vi "LV Demo Main.vi"() -> ()   [LabVIEW 2017, in "Powermeter_library.lvlib"]
uses:
  Powermeter_library.lvlib
  Channel States.ctl
  <vilib>/regexp/Match Regular Expression.xnode
panel:
  out "File Size":i64=76
  in  "Tab Control":enum32{"File", "Page 2"}(tab)
  in  "Filename":string="Run1_Powermeter"
  out "file path":path=path "E:/HVOF - Tests/2017/Recombination/2017-10-04/Run1_Powermeter.tdms"
  in  "base path":path=path "E:/HVOF - Tests/2017/Recombination"
  in  "Group name append":string
  in  "Meas On":bool[](array[boolean])=[TRUE]
  in  "scan again":bool=TRUE
  in  "All Handles":i32[](array[numeric])=[1000]
  in  "Get Lib Ver":bool
  in  "Get Driver Ver":bool
  out "LibVer":i32
  out "DriverVer":string
  out "output cluster":T1
  in  "Reset graph 2":bool
  out "Timestamp offset":dbl
  out "First Data point":bool=TRUE
  out "Power meter 2":cluster{timestamp[], dbl[]}(graph)={[timestamp(3586444920.089349 s since 1904-01-01), timestamp(3586444920.2053604 s since 1904-01-01), timestamp(3586444920.2613664 s since 1904-01-01), timestamp(3586444920.370377 s since 1904-01-01), timestamp(3586444920.479388 s since 1904-01-01), timestamp(3586444920.588399 s since 1904-01-01), timestamp(3586444920.70241 s since 1904-01-01), timestamp(3586444920.7584157 s since 1904-01-01), timestamp(3586444920.868427 s since 1904-01-01), timestamp(3586444920.978438 s since 1904-01-01), timestamp(3586444921.0864487 s since 1904-01-01), timestamp(3586444921.19646 s since 1904-01-01), timestamp(3586444921.253465 s since 1904-01-01), timestamp(3586444921.3664765 s since 1904-01-01), timestamp(3586444921.6875086 s since 1904-01-01), timestamp(3586444921.7935195 s since 1904-01-01), timestamp(3586444922.0625463 s since 1904-01-01), timestamp(3586444922.170557 s since 1904-01-01), timestamp(3586444922.491589 s since 1904-01-01), timestamp(3586444922.6016 s since 1904-01-01), timestamp(3586444922.868627 s since 1904-01-01), timestamp(3586444922.977638 s since 1904-01-01), timestamp(3586444923.29867 s since 1904-01-01), timestamp(3586444923.3546753 s since 1904-01-01), timestamp(3586444923.6767077 s since 1904-01-01), timestamp(3586444923.7857184 s since 1904-01-01), timestamp(3586444924.0537453 s since 1904-01-01), timestamp(3586444924.161756 s since 1904-01-01), timestamp(3586444924.270767 s since 1904-01-01), timestamp(3586444924.379778 s since 1904-01-01), timestamp(3586444924.489789 s since 1904-01-01), timestamp(3586444924.6028004 s since 1904-01-01), timestamp(3586444924.6558056 s since 1904-01-01), timestamp(3586444924.772817 s since 1904-01-01), timestamp(3586444924.880828 s since 1904-01-01), timestamp(3586444924.952835 s since 1904-01-01), timestamp(3586444925.062846 s since 1904-01-01), timestamp(3586444925.168857 s since 1904-01-01), timestamp(3586444925.2788677 s since 1904-01-01), timestamp(3586444925.3868785 s since 1904-01-01), timestamp(3586444925.4968896 s since 1904-01-01), timestamp(3586444925.552895 s since 1904-01-01), timestamp(3586444925.6619062 s since 1904-01-01), timestamp(3586444925.770917 s since 1904-01-01), timestamp(3586444925.879928 s since 1904-01-01), timestamp(3586444925.987939 s since 1904-01-01), timestamp(3586444926.0939493 s since 1904-01-01), timestamp(3586444926.149955 s since 1904-01-01), timestamp(3586444926.2609663 s since 1904-01-01), timestamp(3586444926.370977 s since 1904-01-01), timestamp(3586444926.479988 s since 1904-01-01), timestamp(3586444926.588999 s since 1904-01-01), timestamp(3586444926.69801 s since 1904-01-01), timestamp(3586444926.7540154 s since 1904-01-01), timestamp(3586444926.863026 s since 1904-01-01), timestamp(3586444926.9760375 s since 1904-01-01), timestamp(3586444927.0850487 s since 1904-01-01), timestamp(3586444927.191059 s since 1904-01-01), timestamp(3586444927.30207 s since 1904-01-01), timestamp(3586444927.356076 s since 1904-01-01), timestamp(3586444927.4650865 s since 1904-01-01), timestamp(3586444927.5790977 s since 1904-01-01), timestamp(3586444927.688109 s since 1904-01-01), timestamp(3586444927.849125 s since 1904-01-01), timestamp(3586444927.9581356 s since 1904-01-01), timestamp(3586444928.0681467 s since 1904-01-01), timestamp(3586444928.180158 s since 1904-01-01), timestamp(3586444928.289169 s since 1904-01-01), timestamp(3586444928.39818 s since 1904-01-01), timestamp(3586444928.4661865 s since 1904-01-01), timestamp(3586444928.581198 s since 1904-01-01), timestamp(3586444928.6942096 s since 1904-01-01), timestamp(3586444928.750215 s since 1904-01-01), timestamp(3586444928.870227 s since 1904-01-01), timestamp(3586444928.9772377 s since 1904-01-01), timestamp(3586444929.0932493 s since 1904-01-01), timestamp(3586444929.149255 s since 1904-01-01), timestamp(3586444929.259266 s since 1904-01-01), timestamp(3586444929.3672767 s since 1904-01-01), timestamp(3586444929.4762874 s since 1904-01-01), timestamp(3586444929.5852985 s since 1904-01-01), timestamp(3586444929.694309 s since 1904-01-01), timestamp(3586444929.750315 s since 1904-01-01), timestamp(3586444929.862326 s since 1904-01-01), timestamp(3586444929.9763374 s since 1904-01-01), timestamp(3586444930.0863485 s since 1904-01-01), timestamp(3586444930.1943593 s since 1904-01-01), timestamp(3586444930.249365 s since 1904-01-01), timestamp(3586444930.358376 s since 1904-01-01), timestamp(3586444930.4763875 s since 1904-01-01), timestamp(3586444930.5853987 s since 1904-01-01), timestamp(3586444930.6944094 s since 1904-01-01), timestamp(3586444930.7514153 s since 1904-01-01), timestamp(3586444930.859426 s since 1904-01-01), timestamp(3586444930.9654365 s since 1904-01-01), timestamp(3586444931.0754476 s since 1904-01-01), timestamp(3586444931.190459 s since 1904-01-01), timestamp(3586444931.29947 s since 1904-01-01), timestamp(3586444931.3554754 s since 1904-01-01), timestamp(3586444931.4644866 s since 1904-01-01), timestamp(3586444931.7845182 s since 1904-01-01), timestamp(3586444931.8935294 s since 1904-01-01), timestamp(3586444931.949535 s since 1904-01-01), timestamp(3586444932.059546 s since 1904-01-01), timestamp(3586444932.1685567 s since 1904-01-01), timestamp(3586444932.277568 s since 1904-01-01), timestamp(3586444932.3875785 s since 1904-01-01), timestamp(3586444932.4965897 s since 1904-01-01), timestamp(3586444932.552595 s since 1904-01-01), timestamp(3586444932.6616063 s since 1904-01-01), timestamp(3586444932.770617 s since 1904-01-01), timestamp(3586444932.8796277 s since 1904-01-01), timestamp(3586444932.9866385 s since 1904-01-01), timestamp(3586444933.0956497 s since 1904-01-01), timestamp(3586444933.151655 s since 1904-01-01), timestamp(3586444933.2616663 s since 1904-01-01), timestamp(3586444933.374677 s since 1904-01-01), timestamp(3586444933.4836884 s since 1904-01-01), timestamp(3586444933.592699 s since 1904-01-01), timestamp(3586444933.649705 s since 1904-01-01), timestamp(3586444933.7587156 s since 1904-01-01), timestamp(3586444933.8667264 s since 1904-01-01), timestamp(3586444933.9757376 s since 1904-01-01), timestamp(3586444934.0837483 s since 1904-01-01), timestamp(3586444934.191759 s since 1904-01-01), timestamp(3586444934.29977 s since 1904-01-01), timestamp(3586444934.3557754 s since 1904-01-01), timestamp(3586444934.4647865 s since 1904-01-01), timestamp(3586444934.573797 s since 1904-01-01), timestamp(3586444934.6828084 s since 1904-01-01), timestamp(3586444934.791819 s since 1904-01-01), timestamp(3586444934.89883 s since 1904-01-01), timestamp(3586444934.9548354 s since 1904-01-01), timestamp(3586444935.063846 s since 1904-01-01), timestamp(3586444935.171857 s since 1904-01-01), timestamp(3586444935.280868 s since 1904-01-01), timestamp(3586444935.3898787 s since 1904-01-01), timestamp(3586444935.49989 s since 1904-01-01), timestamp(3586444935.5568957 s since 1904-01-01), timestamp(3586444935.6659064 s since 1904-01-01), timestamp(3586444935.770917 s since 1904-01-01), timestamp(3586444935.879928 s since 1904-01-01), timestamp(3586444935.988939 s since 1904-01-01), timestamp(3586444936.0979495 s since 1904-01-01), timestamp(3586444936.1539555 s since 1904-01-01), timestamp(3586444936.261966 s since 1904-01-01), timestamp(3586444936.370977 s since 1904-01-01), timestamp(3586444936.479988 s since 1904-01-01), timestamp(3586444936.588999 s since 1904-01-01), timestamp(3586444936.69901 s since 1904-01-01), timestamp(3586444936.7550154 s since 1904-01-01), timestamp(3586444936.864026 s since 1904-01-01), timestamp(3586444936.9720373 s since 1904-01-01), timestamp(3586444937.081048 s since 1904-01-01), timestamp(3586444937.189059 s since 1904-01-01), timestamp(3586444937.29907 s since 1904-01-01), timestamp(3586444937.3550754 s since 1904-01-01), timestamp(3586444937.4640865 s since 1904-01-01), timestamp(3586444937.573097 s since 1904-01-01), timestamp(3586444937.6831083 s since 1904-01-01)], [0.0, 0.0, 0.0, 0.0, 0.0, 0.0, 0.0, 0.0, 0.0, 0.0, 0.0, 0.0, 0.0, 0.0, 0.0, 0.0, 0.0, 0.0, 0.0, 0.0, 0.0, 0.0, 0.0, 0.0, 0.0, 0.0, 0.0, 0.0, 0.0, 0.0, 0.0, 0.0, 0.0, 0.0, 0.0, 0.0, 0.0, 0.0, 0.0, 0.0, 0.0, 0.0, 0.0, 0.0, 0.0, 0.0, 0.0, 0.0, 0.0, 0.0, 0.0, 0.0, 0.0, 0.0, 0.0, 0.0, 0.0, 0.0, 0.0, 0.0, 0.0, 0.0, 0.0, 0.0, 0.0, 0.0, 0.0, 0.0, 0.0, 0.0, 0.0, 0.0, 0.0, 0.0, 0.0, 0.0, 0.0, 0.0, 0.0, 0.0, 0.0, 0.0, 0.0, 0.0, 0.0, 0.0, 0.0, 0.0, 0.0, 0.0, 0.0, 0.0, 0.0, 0.0, 0.0, 0.0, 0.0, 0.0, 0.0, 0.0, 0.0, 0.0, 0.0, 0.0, 0.0, 0.0, 0.0, 0.0, 0.0, 0.0, 0.0, 0.0, 0.0, 0.0, 0.0, 0.0, 0.0, 0.0, 0.0, 0.0, 0.0, 0.0, 0.0, 0.0, 0.0, 0.0, 0.0, 0.0, 0.0, 0.0, 0.0, 0.0, 0.0, 0.0, 0.0, 0.0, 0.0, 0.0, 0.0, 0.0, 0.0, 0.0, 0.0, 0.0, 0.0, 0.0, 0.0, 0.0, 0.0, 0.0, 0.0, 0.0, 0.0, 0.0, 0.0, 0.0, 0.0, 0.0, 0.0, 0.0]}
  in  "Reset graph 1":bool
  out "TDMS error":errorcluster
  out "TDMS file":refnum<k34>
  out "Power meter 1":cluster{timestamp[], dbl[]}(graph)={[timestamp(3586444920.089349 s since 1904-01-01), timestamp(3586444920.2053604 s since 1904-01-01), timestamp(3586444920.2613664 s since 1904-01-01), timestamp(3586444920.370377 s since 1904-01-01), timestamp(3586444920.479388 s since 1904-01-01), timestamp(3586444920.588399 s since 1904-01-01), timestamp(3586444920.70241 s since 1904-01-01), timestamp(3586444920.7584157 s since 1904-01-01), timestamp(3586444920.868427 s since 1904-01-01), timestamp(3586444920.978438 s since 1904-01-01), timestamp(3586444921.0864487 s since 1904-01-01), timestamp(3586444921.19646 s since 1904-01-01), timestamp(3586444921.253465 s since 1904-01-01), timestamp(3586444921.3664765 s since 1904-01-01), timestamp(3586444921.6875086 s since 1904-01-01), timestamp(3586444921.7935195 s since 1904-01-01), timestamp(3586444922.0625463 s since 1904-01-01), timestamp(3586444922.170557 s since 1904-01-01), timestamp(3586444922.491589 s since 1904-01-01), timestamp(3586444922.6016 s since 1904-01-01), timestamp(3586444922.868627 s since 1904-01-01), timestamp(3586444922.977638 s since 1904-01-01), timestamp(3586444923.29867 s since 1904-01-01), timestamp(3586444923.3546753 s since 1904-01-01), timestamp(3586444923.6767077 s since 1904-01-01), timestamp(3586444923.7857184 s since 1904-01-01), timestamp(3586444924.0537453 s since 1904-01-01), timestamp(3586444924.161756 s since 1904-01-01), timestamp(3586444924.270767 s since 1904-01-01), timestamp(3586444924.379778 s since 1904-01-01), timestamp(3586444924.489789 s since 1904-01-01), timestamp(3586444924.6028004 s since 1904-01-01), timestamp(3586444924.6558056 s since 1904-01-01), timestamp(3586444924.772817 s since 1904-01-01), timestamp(3586444924.880828 s since 1904-01-01), timestamp(3586444924.952835 s since 1904-01-01), timestamp(3586444925.062846 s since 1904-01-01), timestamp(3586444925.168857 s since 1904-01-01), timestamp(3586444925.2788677 s since 1904-01-01), timestamp(3586444925.3868785 s since 1904-01-01), timestamp(3586444925.4968896 s since 1904-01-01), timestamp(3586444925.552895 s since 1904-01-01), timestamp(3586444925.6619062 s since 1904-01-01), timestamp(3586444925.770917 s since 1904-01-01), timestamp(3586444925.879928 s since 1904-01-01), timestamp(3586444925.987939 s since 1904-01-01), timestamp(3586444926.0939493 s since 1904-01-01), timestamp(3586444926.149955 s since 1904-01-01), timestamp(3586444926.2609663 s since 1904-01-01), timestamp(3586444926.370977 s since 1904-01-01), timestamp(3586444926.479988 s since 1904-01-01), timestamp(3586444926.588999 s since 1904-01-01), timestamp(3586444926.69801 s since 1904-01-01), timestamp(3586444926.7540154 s since 1904-01-01), timestamp(3586444926.863026 s since 1904-01-01), timestamp(3586444926.9760375 s since 1904-01-01), timestamp(3586444927.0850487 s since 1904-01-01), timestamp(3586444927.191059 s since 1904-01-01), timestamp(3586444927.30207 s since 1904-01-01), timestamp(3586444927.356076 s since 1904-01-01), timestamp(3586444927.4650865 s since 1904-01-01), timestamp(3586444927.5790977 s since 1904-01-01), timestamp(3586444927.688109 s since 1904-01-01), timestamp(3586444927.849125 s since 1904-01-01), timestamp(3586444927.9581356 s since 1904-01-01), timestamp(3586444928.0681467 s since 1904-01-01), timestamp(3586444928.180158 s since 1904-01-01), timestamp(3586444928.289169 s since 1904-01-01), timestamp(3586444928.39818 s since 1904-01-01), timestamp(3586444928.4661865 s since 1904-01-01), timestamp(3586444928.581198 s since 1904-01-01), timestamp(3586444928.6942096 s since 1904-01-01), timestamp(3586444928.750215 s since 1904-01-01), timestamp(3586444928.870227 s since 1904-01-01), timestamp(3586444928.9772377 s since 1904-01-01), timestamp(3586444929.0932493 s since 1904-01-01), timestamp(3586444929.149255 s since 1904-01-01), timestamp(3586444929.259266 s since 1904-01-01), timestamp(3586444929.3672767 s since 1904-01-01), timestamp(3586444929.4762874 s since 1904-01-01), timestamp(3586444929.5852985 s since 1904-01-01), timestamp(3586444929.694309 s since 1904-01-01), timestamp(3586444929.750315 s since 1904-01-01), timestamp(3586444929.862326 s since 1904-01-01), timestamp(3586444929.9763374 s since 1904-01-01), timestamp(3586444930.0863485 s since 1904-01-01), timestamp(3586444930.1943593 s since 1904-01-01), timestamp(3586444930.249365 s since 1904-01-01), timestamp(3586444930.358376 s since 1904-01-01), timestamp(3586444930.4763875 s since 1904-01-01), timestamp(3586444930.5853987 s since 1904-01-01), timestamp(3586444930.6944094 s since 1904-01-01), timestamp(3586444930.7514153 s since 1904-01-01), timestamp(3586444930.859426 s since 1904-01-01), timestamp(3586444930.9654365 s since 1904-01-01), timestamp(3586444931.0754476 s since 1904-01-01), timestamp(3586444931.190459 s since 1904-01-01), timestamp(3586444931.29947 s since 1904-01-01), timestamp(3586444931.3554754 s since 1904-01-01), timestamp(3586444931.4644866 s since 1904-01-01), timestamp(3586444931.7845182 s since 1904-01-01), timestamp(3586444931.8935294 s since 1904-01-01), timestamp(3586444931.949535 s since 1904-01-01), timestamp(3586444932.059546 s since 1904-01-01), timestamp(3586444932.1685567 s since 1904-01-01), timestamp(3586444932.277568 s since 1904-01-01), timestamp(3586444932.3875785 s since 1904-01-01), timestamp(3586444932.4965897 s since 1904-01-01), timestamp(3586444932.552595 s since 1904-01-01), timestamp(3586444932.6616063 s since 1904-01-01), timestamp(3586444932.770617 s since 1904-01-01), timestamp(3586444932.8796277 s since 1904-01-01), timestamp(3586444932.9866385 s since 1904-01-01), timestamp(3586444933.0956497 s since 1904-01-01), timestamp(3586444933.151655 s since 1904-01-01), timestamp(3586444933.2616663 s since 1904-01-01), timestamp(3586444933.374677 s since 1904-01-01), timestamp(3586444933.4836884 s since 1904-01-01), timestamp(3586444933.592699 s since 1904-01-01), timestamp(3586444933.649705 s since 1904-01-01), timestamp(3586444933.7587156 s since 1904-01-01), timestamp(3586444933.8667264 s since 1904-01-01), timestamp(3586444933.9757376 s since 1904-01-01), timestamp(3586444934.0837483 s since 1904-01-01), timestamp(3586444934.191759 s since 1904-01-01), timestamp(3586444934.29977 s since 1904-01-01), timestamp(3586444934.3557754 s since 1904-01-01), timestamp(3586444934.4647865 s since 1904-01-01), timestamp(3586444934.573797 s since 1904-01-01), timestamp(3586444934.6828084 s since 1904-01-01), timestamp(3586444934.791819 s since 1904-01-01), timestamp(3586444934.89883 s since 1904-01-01), timestamp(3586444934.9548354 s since 1904-01-01), timestamp(3586444935.063846 s since 1904-01-01), timestamp(3586444935.171857 s since 1904-01-01), timestamp(3586444935.280868 s since 1904-01-01), timestamp(3586444935.3898787 s since 1904-01-01), timestamp(3586444935.49989 s since 1904-01-01), timestamp(3586444935.5568957 s since 1904-01-01), timestamp(3586444935.6659064 s since 1904-01-01), timestamp(3586444935.770917 s since 1904-01-01), timestamp(3586444935.879928 s since 1904-01-01), timestamp(3586444935.988939 s since 1904-01-01), timestamp(3586444936.0979495 s since 1904-01-01), timestamp(3586444936.1539555 s since 1904-01-01), timestamp(3586444936.261966 s since 1904-01-01), timestamp(3586444936.370977 s since 1904-01-01), timestamp(3586444936.479988 s since 1904-01-01), timestamp(3586444936.588999 s since 1904-01-01), timestamp(3586444936.69901 s since 1904-01-01), timestamp(3586444936.7550154 s since 1904-01-01), timestamp(3586444936.864026 s since 1904-01-01), timestamp(3586444936.9720373 s since 1904-01-01), timestamp(3586444937.081048 s since 1904-01-01), timestamp(3586444937.189059 s since 1904-01-01), timestamp(3586444937.29907 s since 1904-01-01), timestamp(3586444937.3550754 s since 1904-01-01), timestamp(3586444937.4640865 s since 1904-01-01), timestamp(3586444937.573097 s since 1904-01-01), timestamp(3586444937.6831083 s since 1904-01-01)], [0.0, 0.0, 0.0, 0.0, 0.0, 0.0, 0.0, 0.0, 0.0, 0.0, 0.0, 0.0, 0.0, 0.0, 0.0, 0.0, 0.0, 0.0, 0.0, 0.0, 0.0, 0.0, 0.0, 0.0, 0.0, 0.0, 0.0, 0.0, 0.0, 0.0, 0.0, 0.0, 0.0, 0.0, 0.0, 0.0, 0.0, 0.0, 0.0, 0.0, 0.0, 0.0, 0.0, 0.0, 0.0, 0.0, 0.0, 0.0, 0.0, 0.0, 0.0, 0.0, 0.0, 0.0, 0.0, 0.0, 0.0, 0.0, 0.0, 0.0, 0.0, 0.0, 0.0, 0.0, 0.0, 0.0, 0.0, 0.0, 0.0, 0.0, 0.0, 0.0, 0.0, 0.0, 0.0, 0.0, 0.0, 0.0, 0.0, 0.0, 0.0, 0.0, 0.0, 0.0, 0.0, 0.0, 0.0, 0.0, 0.0, 0.0, 0.0, 0.0, 0.0, 0.0, 0.0, 0.0, 0.0, 0.0, 0.0, 0.0, 0.0, 0.0, 0.0, 0.0, 0.0, 0.0, 0.0, 0.0, 0.0, 0.0, 0.0, 0.0, 0.0, 0.0, 0.0, 0.0, 0.0, 0.0, 0.0, 0.0, 0.0, 0.0, 0.0, 0.0, 0.0, 0.0, 0.0, 0.0, 0.0, 0.0, 0.0, 0.0, 0.0, 0.0, 0.0, 0.0, 0.0, 0.0, 0.0, 0.0, 0.0, 0.0, 0.0, 0.0, 0.0, 0.0, 0.0, 0.0, 0.0, 0.0, 0.0, 0.0, 0.0, 0.0, 0.0, 0.0, 0.0, 0.0, 0.0, 0.0]}
  in  "Save data":bool=TRUE
  in  "Stop":bool
  out "ReadStr":string
  in  "Read/Write":T2
  out "Device Name":string="(0)"
  in  "Dev Control":T3 {"externTrigModes" items=["Rising Edge", "Falling Edge", "High Level", "Low Level", "Output High", "Output Low"]; "Stream Modes:" items=["Turbo", "Turbo Freq", "Immediate"]}
  out "Last Error Code:":string="No Error"
  in  "Gen'l Ops":T4
  # "Local variables"
  # "v1.14"
  # "Write / Read"
  # "Device Control"
  # "Streams:"
  # "Ext Trig::"
  # "Device Management"
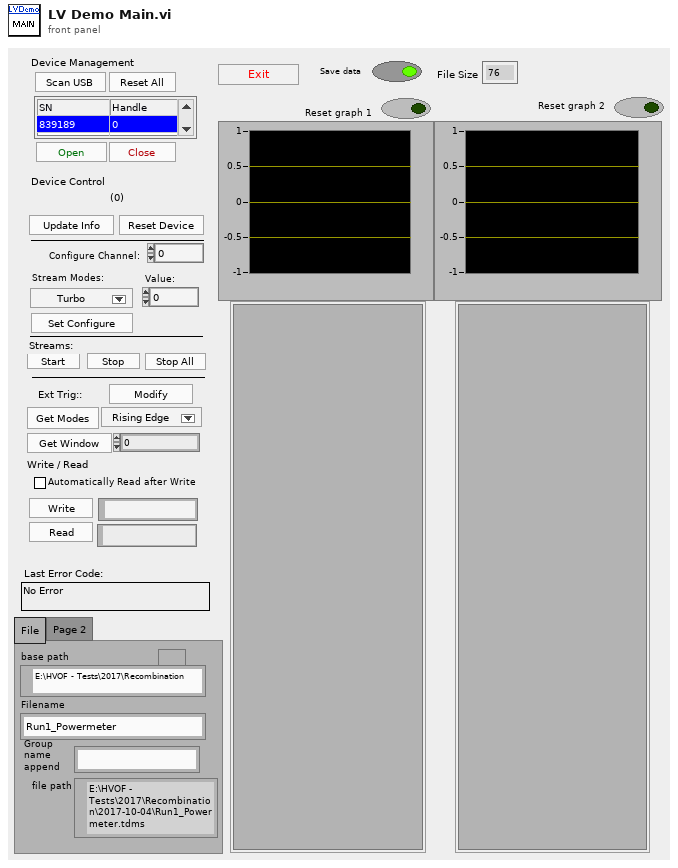
[diagram p1: front panel]
types:
  T1 = cluster{"output cluster 2":cluster{"Value:":dbl[], timestamp[], string[][]}, "output cluster 3":cluster{"Value:":dbl[], timestamp[], string[][]}}
  T2 = cluster{"AutoRead":bool, "Write":bool, "Read":bool, "WriteStr":string}
  T3 = cluster{"UpdateInfo":bool, "ResetDev":bool, "ConfigCh":i32, "Stream Modes:":i32, "Value":i32, "SetConfig":bool, "StartStream":bool, "StopStream":bool, "StopAll":bool, "externTrigModes":i32, "GetModes":bool, "GetWindow":bool, "ExtTrig Window":i32, "Modify":bool}
  T4 = cluster{"scanUSB":bool, "Devices":i32, "Open":bool, "Close":bool, "ResetAll":bool}
  T5 = cluster{"Value:":dbl[], " Time:":string[], " Status:":string[]}
  T6 = enum32{"invalid app kind", "Development System", "Run Time System", "Student Edition", "Embedded LabVIEW", "Evaluation", "Custom"}
  T7 = cluster{"Value:":dbl[], " Time:":string[], " Status:":string[]}[]
  T8 = typedef "Powermeter_library.lvlib/Channel States.ctl" = enum16{"Init", "Poll", "Set Handle", "Measure"}
  T9 = enum16{"open", "open or create", "create or replace", "create", "open (read-only)"}
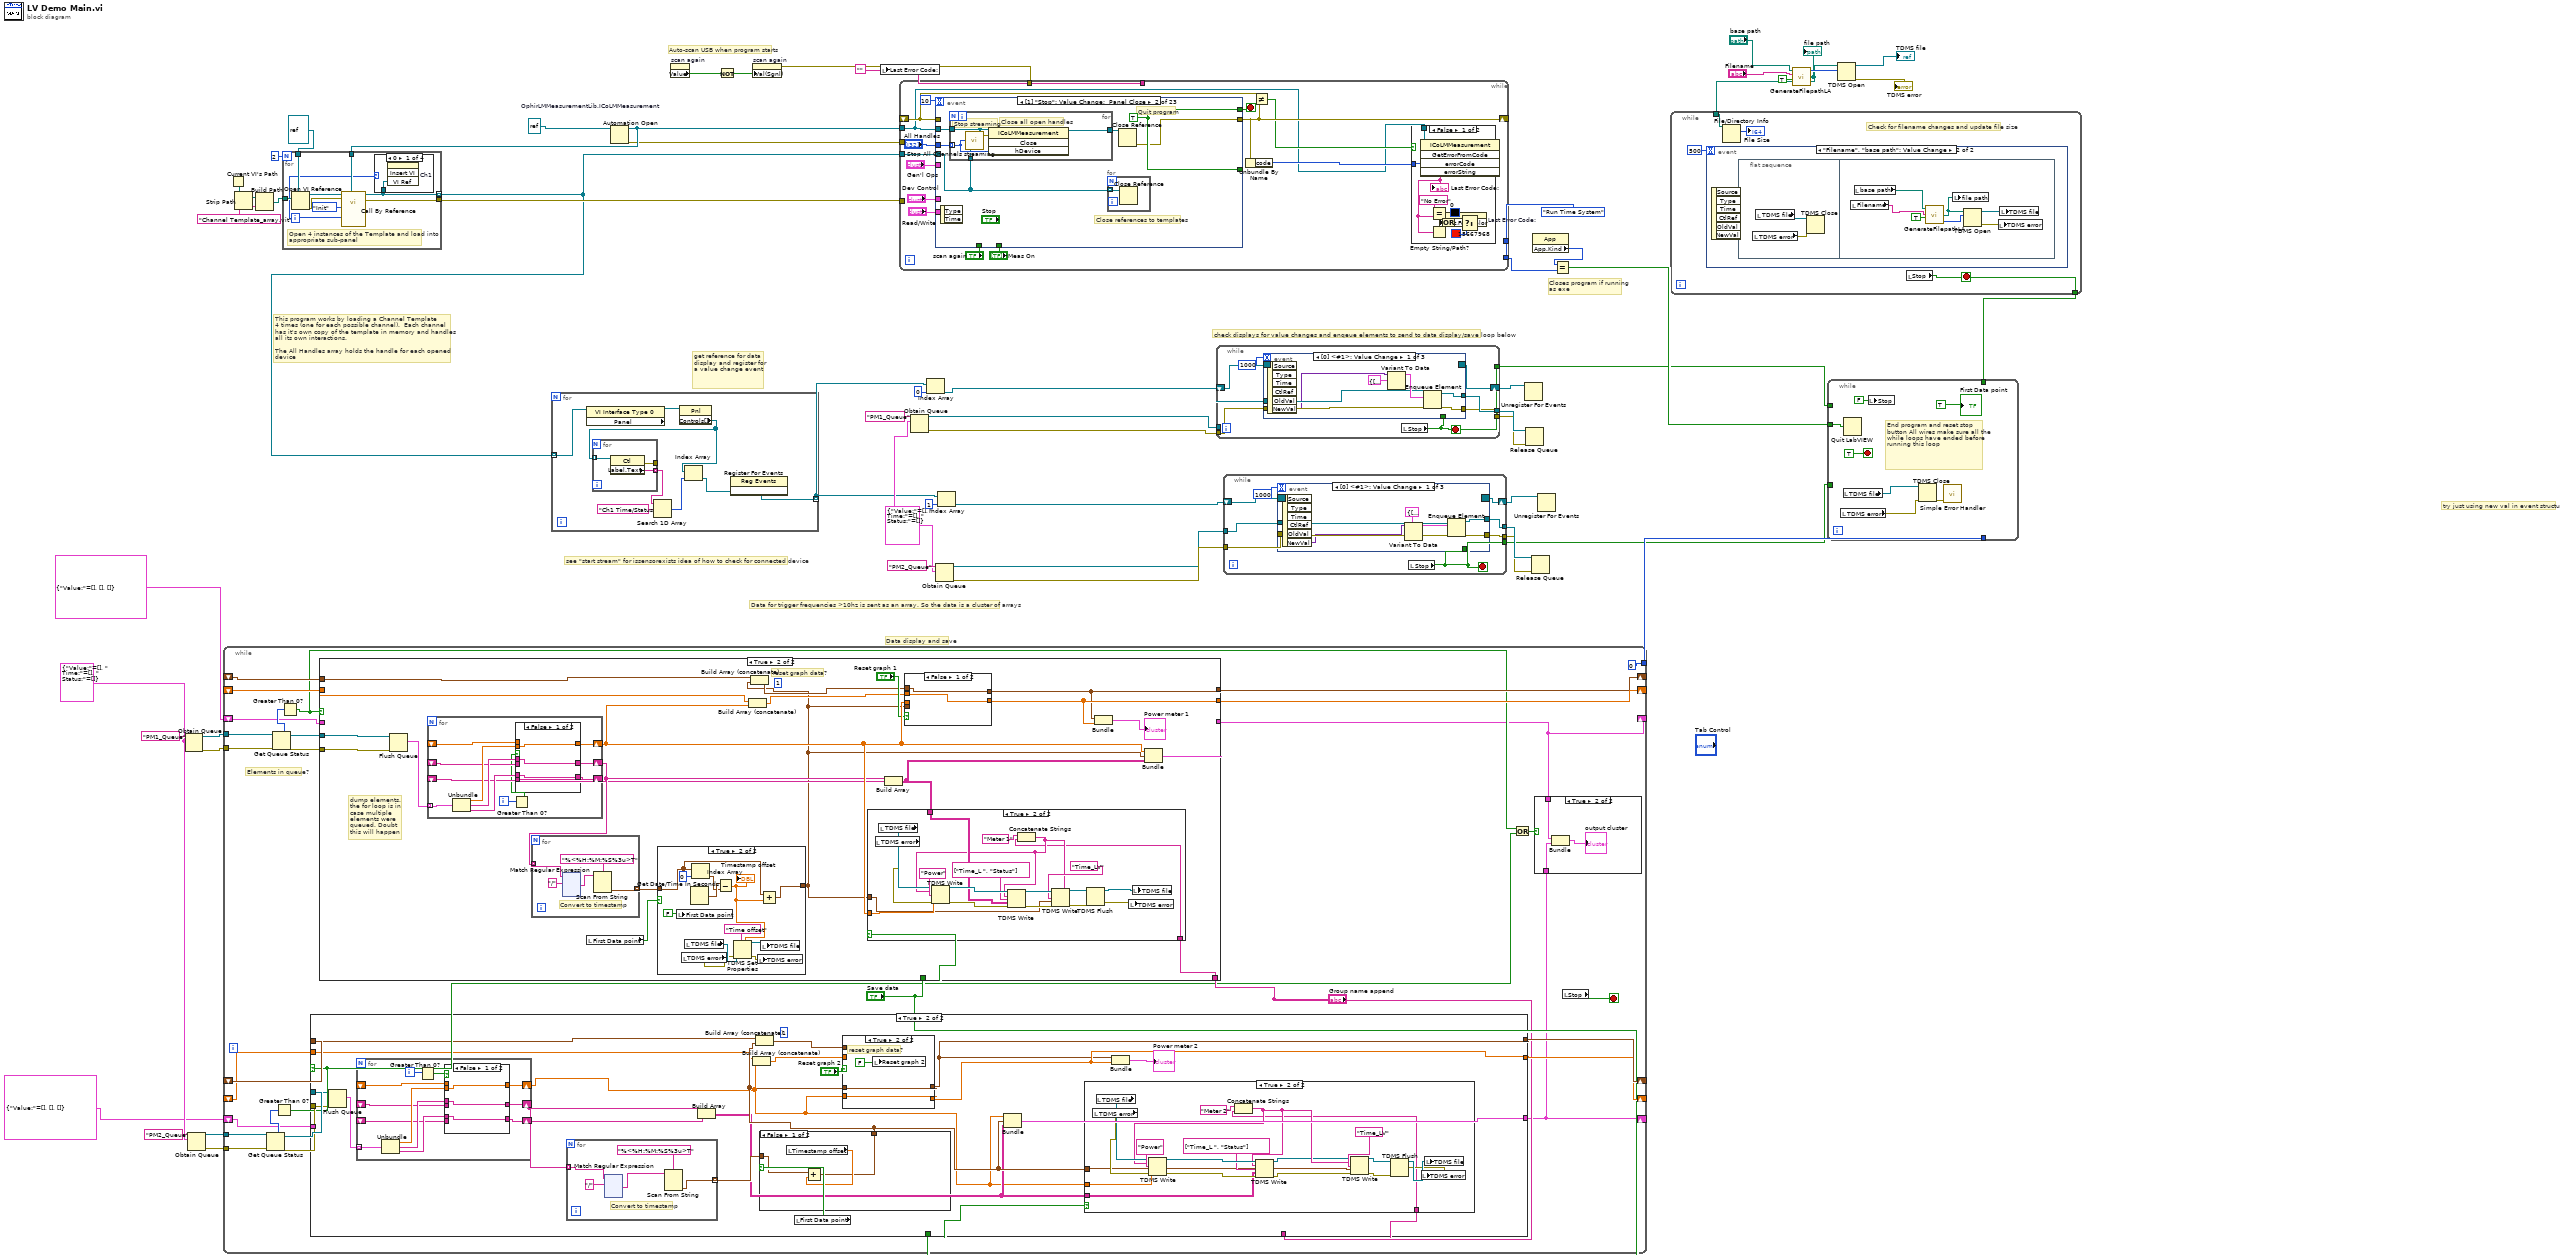
[diagram p0: block diagram]
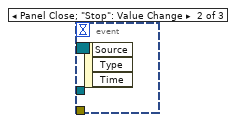
[diagram p2: hidden frame]
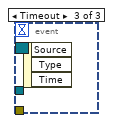
[diagram p3: hidden frame]
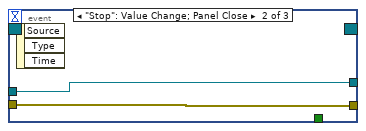
[diagram p4: hidden frame]
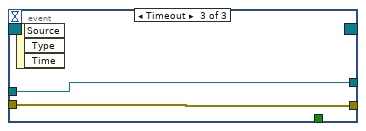
[diagram p5: hidden frame]
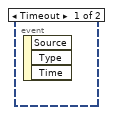
[diagram p6: hidden frame]
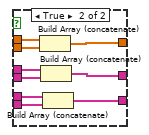
[diagram p9: hidden frame]
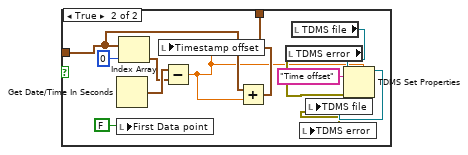
[diagram p11: hidden frame]
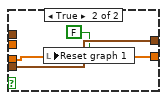
[diagram p14: hidden frame]
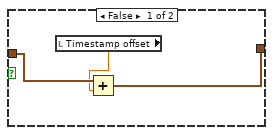
[diagram p15: hidden frame]
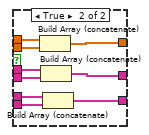
[diagram p17: hidden frame]
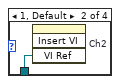
[diagram p18: hidden frame]
diagram:
  w24 = T5 {"Value:"=[], " Time:"=[], " Status:"=[]} ("Ch1 Time/Status")
  w25 = T5 {"Value:"=[], " Time:"=[], " Status:"=[]} ("Ch1 Time/Status")
  w46 = ""
  w57 = refnum<k7> refnum  # OphirLMMeasurementLib.ICoLMMeasurement
  # "Data for trigger frequencies >10hz is sent as an array. So the data is a cluster of arrays"
  # "Data display and save"
  # "check displays for value changes and enqeue elements to send to data display/save loop below"
  # "get reference for data display and register for a value change event"
  # "see \"start stream\" for issensorexists idea of how to check for connected device"
  # "try just using new val in event structure"
  # "Closes program if running\nas exe"
  # "This program works by loading a Channel Template\n4 times (one for each possible channel).  Each channel\nhas it's own copy of the template in memory and handles\nall its own interactions. \n\nThe All Handles array holds the handle for each opened device"
  # "Auto-scan USB when program starts"
  n1 = Obtain Queue(name (unnamed)="PM1_Queue", element data type=w24) -> (queue out=w29:refnum<queue>, error out=w28:errorcluster)  [unwired: 3 in, 1 out]
  n2 = Obtain Queue(name (unnamed)="PM2_Queue", element data type=w24) -> (queue out=w4:refnum<queue>, error out=w3:errorcluster)  [unwired: 3 in, 1 out]
  n3 = while {
    tunnel: [0] -> w39
    shift-right: [w83] -> _
    shift-left: _ -> [w84]
    shift-right: [w82] -> _
    shift-left: _ -> [w85]
    tunnel: w29 -> [w79]
    tunnel: w28 -> [w80]
    tunnel: w4 -> [w72]
    tunnel: w3 -> [w71]
    shift-right: [w70] -> _
    shift-left: _ -> [w68]
    shift-right: [w69] -> _
    shift-left: _ -> [w67]
    shift-right: [w64] -> _
    shift-left: cluster{"Value:":dbl[], timestamp[], string[][]} {"Value:"=[], [], []} ("output cluster 3") -> [w60]
    shift-right: [w59] -> _
    shift-left: cluster{"Value:":dbl[], timestamp[], string[][]} {"Value:"=[], [], []} ("output cluster 2") -> [w58]
    stop <- w86 stop-if-true
    # "Elements in queue?"
    n4 = Get Queue Status(queue=w72, error in (no error)=w71) -> (queue out=w74:refnum<queue>, error out=w73:errorcluster, # elements in queue=w75:i32)  [unwired: 1 in, 5 out]
    n5 = Get Queue Status(queue=w79, error in (no error)=w80) -> (queue out=w77:refnum<queue>, error out=w76:errorcluster, # elements in queue=w78:i32)  [unwired: 1 in, 5 out]
    n6 = Greater Than 0?(x=w75) -> (x > 0?=w62:bool)
    n7 = Greater Than 0?(x=w78) -> (x > 0?=w61:bool)
    n8 = case shown="True" w62 {
      tunnel: w68 -> [w91 w113]
      tunnel: w67 -> [w92 w97]
      tunnel: [w92 w112] -> w69
      tunnel: [w91 w111] -> w70
      tunnel: w74 -> [_ w110]
      tunnel: w73 -> [_ w109]
      tunnel: "Save data" -> [_ w108]
      tunnel: "Group name append" -> [_ w107]
      tunnel: [w90 w106] -> w64
      tunnel: w60 -> [w90 _]
      frame False {
      }
      frame True {
        (unwired) 1
        n9 = Flush Queue(queue=w110, error in (no error)=w109) -> (remaining elements=w96:T7)  [unwired: 2 out]
        n10 = for {
          tunnel: w96 -> [w125] mode=indexing
          shift-right: [w123] -> w93
          shift-left: _ -> [w122]
          shift-right: [w119] -> w95
          shift-left: _ -> [w118]
          shift-right: [w117] -> w94
          shift-left: _ -> [w116]
          i -> [w115]
          n11 = Unbundle(w125) -> ("Value:"=w124:dbl[], "Time:"=w121:string[], "Status:"=w120:string[])
          n12 = Greater Than 0?(x=w115) -> (x > 0?=w114:bool)
          n13 = case shown="False" w114 {
            tunnel: w124 -> [w128 w137]
            tunnel: [w128 w136] -> w123
            tunnel: w122 -> [_ w135]
            tunnel: w121 -> [w127 w134]
            tunnel: w120 -> [w126 w133]
            tunnel: [w127 w132] -> w119
            tunnel: w118 -> [_ w131]
            tunnel: [w126 w130] -> w117
            tunnel: w116 -> [_ w129]
            frame False {
            }
            frame True {
              n14 = Build Array (concatenate)(w135, w137) -> (w136:dbl[])
              n15 = Build Array (concatenate)(w134, w131) -> (w132:string[])
              n16 = Build Array (concatenate)(w133, w129) -> (w130:string[])
            }
          }
        }
        n17 = for {
          tunnel: w95 -> [w160] mode=indexing
          tunnel: [w161] -> w103 mode=indexing
          # "Convert to timestamp"
          n18 = xnode "Match Regular Expression"("input string"=w160, "regular expression"="/") -> ("after match"=w159:string)  [unwired: 4 in, 4 out]
          n19 = Scan From String(format string="%<%H:%M:%S%3u>T", input string=w159) -> (output 1=w161:timestamp)  [unwired: 3 in, 3 out]
        }
        n20 = Build Array(w95, w94) -> (w98:string[][])
        n21 = Build Array (concatenate)(w97, w93) -> (w101:dbl[])
        n22 = local read "First Data point"() -> (w104:bool)
        n23 = case shown="False" w104 {
          tunnel: w103 -> [w145 w153]
          tunnel: [w143 w152] -> w99
          frame False {
            n24 = local read "Timestamp offset"() -> (w144:dbl)
            n25 = Add(x=w145, y=w144) -> (x+y=w143:timestamp[])
          }
          frame True {
            n26 = Get Date/Time In Seconds() -> (seconds since 1Jan1904=w156:timestamp)
            n27 = local write "First Data point"(FALSE) -> ()
            n28 = Index Array(array=w153, index=0) -> (element=w155:timestamp)
            n29 = Subtract(x=w156, y=w155) -> (x-y=w148:dbl)
            n30 = local write "Timestamp offset"(w148) -> ()
            n31 = Add(x=w153, y=w148) -> (x+y=w152:timestamp[])
            n32 = local read "TDMS error"() -> (w150:errorcluster)
            n33 = local read "TDMS file"() -> (w151:refnum<k34>)
            n34 = TDMS Set Properties(5:w148, 7:"Time offset" ("property names"), 8:w150, 11:w151) -> (0:w146:errorcluster, 3:w147:refnum<k34>)  [unwired: 2 in, 2 out]
            n35 = local write "TDMS error"(w146) -> ()
            n36 = local write "TDMS file"(w147) -> ()
          }
        }
        n37 = Build Array (concatenate)(w113, w99) -> (w100:timestamp[])
        n38 = case shown="True" "Reset graph 2" {
          tunnel: w99 -> [_ w142]
          tunnel: w93 -> [_ w141]
          tunnel: [w139 w142] -> w111
          tunnel: [w138 w141] -> w112
          tunnel: w101 -> [w138 _]
          tunnel: w100 -> [w139 _]
          frame False {
          }
          frame True {
            # "reset graph data?"
            n39 = local write "Reset graph 2"(FALSE) -> ()
          }
        }
        n40 = Bundle("Value:"=w93, w99, w98) -> (w106:cluster{"Value:":dbl[], timestamp[], string[][]})  [unwired: 1 in]
        n41 = case shown="True" w108 {
          tunnel: w99 -> [_ w279]
          tunnel: w93 -> [_ w280]
          tunnel: w98 -> [_ w292]
          tunnel: w107 -> [_ w281]
          frame False {
          }
          frame True {
            n42 = local read "TDMS error"() -> (w288:errorcluster)
            n43 = local read "TDMS file"() -> (w289:refnum<k34>)
            n44 = Concatenate Strings("Meter 2", w281) -> (w282:string)
            n45 = TDMS Write(0:w289, 5:w282, 7:"Power", 9:w280, 11:w288) -> (4:w294:refnum<k34>, 15:w293:errorcluster)  [unwired: 1 in, 2 out]
            n46 = TDMS Write(0:w294, 5:w282, 7:string[] ["Time_L ", "Status"], 9:w292, 11:w293) -> (4:w278:refnum<k34>, 15:w277:errorcluster)  [unwired: 1 in, 2 out]
            n47 = TDMS Write(0:w278, 5:w282, 7:"Time_LV", 9:w279, 11:w277) -> (4:w287:refnum<k34>, 15:w286:errorcluster)  [unwired: 1 in, 2 out]
            n48 = TDMS Flush(4:w286, 7:w287) -> (0:w284:errorcluster, 3:w285:refnum<k34>)
            n49 = local write "TDMS error"(w284) -> ()
            n50 = local write "TDMS file"(w285) -> ()
          }
        }
        n51 = Bundle(w111, "Value:"=w112) -> (→"Power meter 2":cluster{timestamp[], "Value:":dbl[]})  [unwired: 1 in]
      }
    }
    n52 = case shown="True" w61 {
      tunnel: w85 -> [w297 w319]
      tunnel: w84 -> [w298 w318]
      tunnel: [w298 w317] -> w83
      tunnel: [w297 w316] -> w82
      tunnel: w77 -> [_ w315]
      tunnel: w76 -> [_ w314]
      tunnel: "Save data" -> [_ w313]
      tunnel: "Group name append" -> [_ w312]
      tunnel: [w296 w311] -> w59
      tunnel: w58 -> [w296 _]
      frame False {
      }
      frame True {
        (unwired) 1
        # "reset graph data?"
        # "dump elements. the for loop is in case multiple elements were queued. Doubt this will happen"
        n53 = Flush Queue(queue=w315, error in (no error)=w314) -> (remaining elements=w299:T7)  [unwired: 2 out]
        n54 = for {
          tunnel: w299 -> [w489] mode=indexing
          shift-right: [w487] -> w310
          shift-left: _ -> [w486]
          shift-right: [w483] -> w309
          shift-left: _ -> [w482]
          shift-right: [w481] -> w308
          shift-left: _ -> [w480]
          i -> [w479]
          n55 = Unbundle(w489) -> ("Value:"=w488:dbl[], "Time:"=w485:string[], "Status:"=w484:string[])
          n56 = Greater Than 0?(x=w479) -> (x > 0?=w478:bool)
          n57 = case shown="False" w478 {
            tunnel: w488 -> [w492 w501]
            tunnel: [w492 w500] -> w487
            tunnel: w486 -> [_ w499]
            tunnel: w485 -> [w491 w498]
            tunnel: w484 -> [w490 w497]
            tunnel: [w491 w496] -> w483
            tunnel: w482 -> [_ w495]
            tunnel: [w490 w494] -> w481
            tunnel: w480 -> [_ w493]
            frame False {
            }
            frame True {
              n58 = Build Array (concatenate)(w499, w501) -> (w500:dbl[])
              n59 = Build Array (concatenate)(w498, w495) -> (w496:string[])
              n60 = Build Array (concatenate)(w497, w493) -> (w494:string[])
            }
          }
        }
        n61 = for {
          tunnel: w309 -> [w342] mode=indexing
          tunnel: [w343] -> w305 mode=indexing
          # "Convert to timestamp"
          n62 = xnode "Match Regular Expression"("input string"=w342, "regular expression"="/") -> ("after match"=w340:string)  [unwired: 4 in, 4 out]
          n63 = Scan From String(format string="%<%H:%M:%S%3u>T", input string=w340) -> (output 1=w343:timestamp)  [unwired: 3 in, 3 out]
        }
        n64 = local read "First Data point"() -> (w306:bool)
        n65 = case shown="True" w306 {
          tunnel: w305 -> [w327 w335]
          tunnel: [w325 w334] -> w301
          frame False {
            n66 = local read "Timestamp offset"() -> (w326:dbl)
            n67 = Add(x=w327, y=w326) -> (x+y=w325:timestamp[])
          }
          frame True {
            n68 = local write "First Data point"(FALSE) -> ()
            n69 = local read "TDMS error"() -> (w330:errorcluster)
            n70 = local read "TDMS file"() -> (w332:refnum<k34>)
            n71 = Get Date/Time In Seconds() -> (seconds since 1Jan1904=w338:timestamp)
            n72 = Index Array(array=w335, index=0) -> (element=w337:timestamp)
            n73 = Subtract(x=w338, y=w337) -> (x-y=w331:dbl)
            "Timestamp offset" <- w331
            n74 = TDMS Set Properties(5:w331, 7:"Time offset" ("property names"), 8:w330, 11:w332) -> (0:w329:errorcluster, 3:w328:refnum<k34>)  [unwired: 2 in, 2 out]
            n75 = local write "TDMS error"(w329) -> ()
            n76 = Add(x=w335, y=w331) -> (x+y=w334:timestamp[])
            n77 = local write "TDMS file"(w328) -> ()
          }
        }
        n78 = Build Array (concatenate)(w318, w310) -> (w303:dbl[])
        n79 = Build Array (concatenate)(w319, w301) -> (w302:timestamp[])
        n80 = Build Array(w309, w308) -> (w300:string[][])
        n81 = case shown="True" w313 {
          tunnel: w301 -> [_ w459]
          tunnel: w310 -> [_ w460]
          tunnel: w300 -> [_ w474]
          tunnel: w312 -> [_ w461]
          frame False {
          }
          frame True {
            n82 = local read "TDMS error"() -> (w468:errorcluster)
            n83 = local read "TDMS file"() -> (w469:refnum<k34>)
            n84 = Concatenate Strings("Meter 1", w461) -> (w462:string)
            n85 = TDMS Write(0:w469, 5:w462, 7:"Power", 9:w460, 11:w468) -> (4:w476:refnum<k34>, 15:w475:errorcluster)  [unwired: 1 in, 2 out]
            n86 = TDMS Write(0:w476, 5:w462, 7:string[] ["Time_L ", "Status"], 9:w474, 11:w475) -> (4:w472:refnum<k34>, 15:w471:errorcluster)  [unwired: 1 in, 2 out]
            n87 = TDMS Write(0:w472, 5:w462, 7:"Time_LV", 9:w459, 11:w471) -> (4:w467:refnum<k34>, 15:w466:errorcluster)  [unwired: 1 in, 2 out]
            n88 = TDMS Flush(4:w466, 7:w467) -> (0:w464:errorcluster, 3:w465:refnum<k34>)
            n89 = local write "TDMS error"(w464) -> ()
            n90 = local write "TDMS file"(w465) -> ()
          }
        }
        n91 = case shown="False" "Reset graph 1" {
          tunnel: w303 -> [w320 _]
          tunnel: w302 -> [w321 _]
          tunnel: w310 -> [_ w324]
          tunnel: w301 -> [_ w323]
          tunnel: [w320 w324] -> w317
          tunnel: [w321 w323] -> w316
          frame False {
          }
          frame True {
            n92 = local write "Reset graph 1"(FALSE) -> ()
          }
        }
        n93 = Bundle(w316, "Value:"=w317) -> (→"Power meter 1":cluster{timestamp[], "Value:":dbl[]})  [unwired: 1 in]
        n94 = Bundle("Value:"=w310, w301, w300) -> (w311:cluster{"Value:":dbl[], timestamp[], string[][]})  [unwired: 1 in]
      }
    }
    n95 = Or(x=w61, y=w62) -> (x .or. y?=w63:bool)
    n96 = case shown="True" w63 {
      tunnel: w59 -> [_ w89]
      tunnel: w64 -> [_ w87]
      frame False {
      }
      frame True {
        n97 = Bundle("output cluster 2"=w89, "output cluster 3"=w87) -> (→"output cluster":T1)  [unwired: 1 in]
      }
    }
    n98 = local read "Stop"() -> (w86:bool)
  }
  n99 = Current VI's Path() -> (path=w55:path)
  n100 = Strip Path(path=w55) -> (stripped path=w54:path)  [unwired: 1 out]
  n101 = Build Path(base path=w54, name or relative path="Channel Template_array.vit") -> (appended path=w52:path)
  n102 = Automation Open(Automation Refnum=w57) -> (Automation Refnum=w42:refnum<k7>, error out=w41:errorcluster)  [unwired: 1 in, 2 out]
  n103 = for {
    N: 2 -> [_]
    tunnel: w52 -> [w510]
    tunnel: refnum<vi> refnum ("type specifier VI Refnum (for type only)") -> [w509]
    tunnel: w42 -> [w506]
    tunnel: [w502] -> w23 mode=indexing
    tunnel: [w504] -> w50
    i -> [w503]
    # "Open 4 instances of the Template and load into\nappropriate sub-panel"
    n104 = Open VI Reference(type specifier VI Refnum (for type only)=w509, vi path=w510) -> (vi reference=w508:refnum<vi>, error out=w505:errorcluster)  [unwired: 1 in, 3 out]
    n105 = call-by-ref "?"(reference=w508, error in=w505, "OphirLMMeasurementLib.ICoLMMeasurement"=w506, "Ch in"=w503, "State"=Channel_States."Init") -> (reference out=w502:refnum<vi>, error out=w504:errorcluster)  [unwired: 7 in, 1 out]
    n106 = case shown="0" w503 {
      tunnel: w502 -> [w511 w512 _ _]
      frame 0 {
        n107 = invoke on="Ch1" class="SubPnl" method="Insert VI"("VI Ref"=w511) -> ()  [unwired: 3 in, 4 out]
      }
      frame 1, Default {
        n108 = invoke on="Ch2" class="SubPnl" method="Insert VI"("VI Ref"=w512) -> ()  [unwired: 3 in, 4 out]
      }
      frame 2 {
      }
      frame 3 {
      }
    }
  }
  n109 = for {
    tunnel: w23 -> [w519] mode=indexing
    tunnel: [w513] -> w22 mode=indexing
    n110 = property class="VI Interface Type 0"(reference=w519) -> ("Panel"=w520:refnum<vi>)  [unwired: 1 in, 2 out]
    n111 = property class="Pnl"(reference=w520) -> ("Controls[]"=w516:refnum<vi>[])  [unwired: 1 in, 2 out]
    n112 = for {
      tunnel: w516 -> [w523] mode=indexing
      tunnel: [w522] -> w518 mode=indexing
      tunnel: [w521] -> _
      n113 = property class="Ctl"(reference=w523) -> (error out=w521:errorcluster, "Label.Text"=w522:string)  [unwired: 1 in, 1 out]
    }
    n114 = Search 1D Array(1D array=w518, element="Ch1 Time/Status") -> (index of element=w515:i32)  [unwired: 1 in]
    n115 = Index Array(array=w516, index=w515) -> (element=w514:refnum<vi>)
    n116 = register-events(w514) -> (reference out=w513:refnum<event-registration>)  [unwired: 2 in, 1 out]
  }
  n117 = property on="scan again" class="Bool (strict)"() -> ("Value"=w48:bool)  [unwired: 2 in, 2 out]
  n118 = Not(x=w48) -> (.not. x?=w49:bool)
  n119 = property on="scan again" class="Bool (strict)"("Val(Sgnl)"=w49) -> (error out=w47:errorcluster)  [unwired: 2 in, 1 out]
  n120 = local write "Last Error Code:"(w46) -> ()
  n121 = while {
    tunnel: w42 -> [w524]
    tunnel: w41 -> [_]
    tunnel: w23 -> [w532]
    tunnel: w50 -> [_]
    tunnel: w47 -> [_]
    tunnel: w46 -> [_]
    tunnel: [w530] -> w43
    tunnel: T6."Run Time System" ("y") -> [w530]
    shift-right: [w527] -> _
    shift-left: _ -> [w528]
    stop <- w538 stop-if-true
    n122 = event shown="[1] \"Stop\": Value Change;  Panel Close" {
      selector: _ -> [_ _ _ _ _ _ _ _ _ _ _ _ _ _ _ _ _ _ _ _ _ _ _]
      dyn-events: _ -> [_ _ _ _ _ _ _ _ _ _ _ _ _ _ _ _ _ _ _ _ _ _ _]
      timeout: 10 -> [_ _ _ _ _ _ _ _ _ _ _ _ _ _ _ _ _ _ _ _ _ _ _]
      tunnel: [_ w562 _ _ _ _ _ _ _ _ _ _ _ _ _ _ _ _ _ _ _ _ _] -> w538
      tunnel: w524 -> [w551 w565 w575 w581 w599 w611 w623 w632 w657 w678 w692 _ w705 w719 w745 w758 w772 w779 w786 w794 w805 w813 _]
      tunnel: [w549 w560 w573 w580 w596 w603 w622 w634 w652 w673 w684 w697 w704 w709 w744 w749 w767 w774 w781 w789 w796 w815 w819] -> w527
      tunnel: "Gen'l Ops" -> [_ _ _ _ _ w608 w621 _ _ w677 w687 _ w702 w718 w746 _ w771 w778 w785 w793 w804 w818 _]
      tunnel: "All Handles" -> [_ w564 _ _ w591 _ w619 w624 w659 w676 w680 _ w703 w717 w747 w753 w770 w777 w784 w792 w803 w817 _]
      tunnel: "Read/Write" -> [_ _ _ _ _ _ _ _ _ _ _ _ _ _ _ _ _ _ _ _ w801 _ _]
      tunnel: "Dev Control" -> [_ _ _ _ _ _ _ _ _ _ _ _ w701 _ _ _ _ _ _ w788 _ _ _]
      tunnel: w532 -> [w553 w561 _ _ _ w605 _ w628 w656 _ w688 _ _ w715 w743 w756 _ _ _ _ _ _ _]
      tunnel: "scan again" -> [_ _ _ _ _ _ _ w633 _ _ _ _ _ _ _ _ _ _ _ _ _ _ _]
      tunnel: [_ w562 TRUE TRUE TRUE _ _ _ _ _ _ _ _ _ _ _ _ _ _ _ _ _ _] -> _
      tunnel: "Meas On" -> [_ _ _ _ _ _ _ _ w654 _ _ _ _ w713 w740 _ _ _ _ _ _ _ _]
      tunnel: w528 -> [w549 _ _ _ _ _ _ _ w652 _ _ w697 _ _ _ _ _ _ _ _ _ _ w819]
      event Timeout {
        # "Poll each Channel to handle user interactions"
        n123 = event-data() -> ()  [unwired: 2 out]
        n124 = for {
          tunnel: w553 -> [w559] mode=indexing
          tunnel: Channel_States."Poll" ("State") -> [w558]
          tunnel: w551 -> [w557]
          shift-right: [w554] -> _
          shift-left: errorcluster {"status"=FALSE, "code"=0, "source"=""} ("error out") -> [w555]
          n125 = call-by-ref "?"(reference=w559, "OphirLMMeasurementLib.ICoLMMeasurement"=w557, "State"=w558) -> ("error out"=w556:errorcluster)  [unwired: 9 in, 2 out]
          n126 = Merge Errors(w556, w555) -> (w554:errorcluster)
        }
      }
      event "Stop": Value Change; Panel Close {
        w562 = TRUE
        # "Close references to templates"
        # "Quit program"
        n127 = event-data() -> ()  [unwired: 3 out]
        n128 = for {
          tunnel: w565 -> [w567]
          tunnel: w564 -> [w569] mode=indexing
          tunnel: [w570] -> w563
          tunnel: w561 -> [w568]
          # "Stop streaming"
          # "Close all open handles"
          n129 = call "Stop All Channels streaming.vi"("Template Refs"=w568, "Handle"=w569, "LMMeasurementLib.ICoLMMeasurement"=w567) -> ("error out"=w566:errorcluster)
          n130 = invoke class="ICoLMMeasurement" method="Close"(reference=w567, error in=w566, "hDevice"=w569) -> (reference out=w570:refnum<k7>)  [unwired: 1 in, 3 out]
        }
        n131 = for {
          tunnel: w561 -> [w571] mode=indexing
          n132 = Close Reference(reference=w571) -> ()  [unwired: 1 in, 1 out]
        }
        n133 = Close Reference(reference=w563) -> (error out=w560:errorcluster)  [unwired: 1 in]
      }
      event "Get Lib Ver": Value Change {
        # "Get library verson from device"
        n134 = event-data() -> ()  [unwired: 2 out]
        n135 = invoke class="ICoLMMeasurement" method="GetVersion"(reference=w575) -> (error out=w573:errorcluster, "version"=→"LibVer":i32)  [unwired: 3 in, 2 out]
      }
      event "Get Driver Ver": Value Change {
        # "Get Driver Info from device"
        n136 = event-data() -> ()  [unwired: 2 out]
        n137 = invoke class="ICoLMMeasurement" method="GetDriverVersion"(reference=w581) -> (error out=w580:errorcluster, "info"=w579:string)  [unwired: 3 in, 2 out]
        n138 = Match Pattern(string=w579, regular expression="Version ") -> (after substring=→"DriverVer":string)  [unwired: 4 out]
      }
      event "Gen'l Ops.scanUSB", "scan again": Value Change {
        # "Look for all USB devices"
        n139 = event-data() -> ()  [unwired: 2 out]
        n140 = property on="Devices" class="MCListbox (strict)"() -> (error out=w590:errorcluster, "ItemNames"=w589:string[][])  [unwired: 2 in, 1 out]
        n141 = invoke class="ICoLMMeasurement" method="ScanUSB"(reference=w599, error in=w590) -> (error out=w596:errorcluster, "serialNumbers"=w598:variant)  [unwired: 2 in, 2 out]
        n142 = Index Array(array=w589, index (col) #1=0 ("disabled index (col)")) -> (element #1=w588:string[])  [unwired: 3 in, 1 out]
        n143 = Variant To Data(type=string[] [], Variant=w598) -> (data=w585:string[])  [unwired: 1 in, 1 out]
        n144 = call "Get Handles for Scan Devices.vi"("Old Device Names"=w588, "All Handles In"=w591, "New Device Names"=w585) -> ("All Handles Out"=w586:i32[], "# handles"=w592:i32)
        n145 = local write "All Handles"(w586) -> ()
        n146 = Initialize Array(FALSE, w592) -> (w593:bool[])
        n147 = Number To Decimal String(number=w586) -> (decimal integer string=w584:string[])  [unwired: 1 out]
        n148 = local write "Meas On"(w593) -> ()
        n149 = Build Array(w585, w584) -> (w583:string[][])
        n150 = Transpose 2D Array(2D array=w583) -> (transposed array=w582:string[][])
        n151 = property on="Devices" class="MCListbox (strict)"("ItemNames"=w582) -> ()  [unwired: 2 in, 2 out]
      }
      event "Gen'l Ops.Open": Value Change {
        # "When opening a device, send its\nhandle to each channel & store\nhandles in All Handles array"
        # "Open selected device"
        n152 = event-data() -> ()  [unwired: 2 out]
        n153 = property on="Devices" class="MCListbox (strict)"() -> ("ItemNames"=w609:string[][])  [unwired: 2 in, 2 out]
        n154 = Unbundle By Name(w608) -> ("Devices"=w607:i32)
        n155 = Index Array(array=w609, index (row)=w607, index (col)=0 ("disabled index (col)")) -> (element=w610:string)
        n156 = invoke class="ICoLMMeasurement" method="OpenUSBDevice"(reference=w611, "serialNumber"=w610) -> (reference out=w604:refnum<k7>, error out=w603:errorcluster, "hDevice"=w606:i32)  [unwired: 3 in, 2 out]
        n157 = control-ref of="Devices"() -> (w601:refnum<vi>)
        n158 = control-ref of="All Handles"() -> (w600:refnum<vi>)
        n159 = call "Set Handle on Open.vi"("error in"=w603, "All Handles ref"=w600, "hDevice"=w606, "Selected Device"=w607, "Ch refs"=w605, "OphirLMMeasurementLib.ICoLMMeasurement"=w604, "Devices List box ref"=w601) -> ()  [unwired: 3 out]
      }
      event "Gen'l Ops.Close": Value Change {
        # "Close selected device"
        n160 = event-data() -> ()  [unwired: 2 out]
        n161 = Unbundle By Name(w621) -> ("Devices"=w615:i32)
        n162 = Index Array(array=w619, index=w615) -> (element=w620:i32)
        n163 = Replace Array Subset(array=w619, new element=0 ("new element/subarray"), index=w615) -> (w618:i32[])
        n164 = invoke class="ICoLMMeasurement" method="Close"(reference=w623, "hDevice"=w620) -> (error out=w622:errorcluster)  [unwired: 2 in, 3 out]
        n165 = local write "All Handles"(w618) -> ()
        n166 = property on="Devices" class="MCListbox (strict)"() -> ("ItemNames"=w617:string[][])  [unwired: 2 in, 2 out]
        n167 = Replace Array Subset(array=w617, new element="0" ("new element/subarray"), index (row)=w615, index (col)=1 ("new element/subarray")) -> (w616:string[][])
        n168 = property on="Devices" class="MCListbox (strict)"("ItemNames"=w616) -> ()  [unwired: 2 in, 2 out]
      }
      event "Gen'l Ops.ResetAll": Value Change {
        # "This is an artificial method for generating an\nevent so the program will rescan the USB\nport after all devices are closed"
        # "Close all devices"
        n169 = event-data() -> ()  [unwired: 2 out]
        n170 = for {
          tunnel: w624 -> [w638] mode=indexing
          shift-right: [w639] -> w631
          shift-left: w632 -> [w640]
          tunnel: FALSE -> [w637]
          tunnel: Channel_States."Measure" ("State") -> [w636]
          tunnel: w628 -> [w635]
          # "For each device"
          n171 = for {
            shift-right: [w641] -> w639
            shift-left: w640 -> [w641]
            tunnel: w638 -> [w645]
            tunnel: w637 -> [w644]
            tunnel: w636 -> [w643]
            tunnel: w635 -> [w642] mode=indexing
            # "Turn off\nMeasure-\nments"
            # "For each channel"
            n172 = call-by-ref "?"(reference=w642, "Set Meas"=w644, "OphirLMMeasurementLib.ICoLMMeasurement"=w641, "Handle in"=w645, "State"=w643) -> ()  [unwired: 7 in, 3 out]
          }
        }
        n173 = Not(x=w633) -> ()  [unwired: 1 out]
        n174 = Array Size(array=w624) -> (size(s)=w625:i32)
        n175 = invoke class="ICoLMMeasurement" method="ResetAllDevices"(reference=w631) -> (error out=w634:errorcluster)  [unwired: 2 in, 2 out]
        n176 = Initialize Array(0 ("new element/subarray"), w625) -> (w627:i32[])
        n177 = local write "All Handles"(w627) -> ()
      }
      event "Gen'l Ops.Devices": Value Change {
        # "Update Handle to each Channel\n(this will also activate chs 2,3,4 if device\nis Pulsar)"
        # "Device changed, so update handle"
        n178 = event-data() -> ("NewVal"=w649:i32)  [unwired: 1 out]
        n179 = Index Array(array=w659, index=w649) -> (element=w646:i32)
        n180 = Number To Decimal String(number=w646) -> (decimal integer string=w647:string)  [unwired: 1 out]
        n181 = property on="Devices" class="MCListbox (strict)"() -> ("ItemNames"=w651:string[][])  [unwired: 2 in, 2 out]
        n182 = Replace Array Subset(array=w651, new element=w647, index (row)=w649, index (col)=1 ("disabled index (col)")) -> (w650:string[][])
        n183 = Index Array(array=w654, index=w649) -> (element=w653:bool)
        n184 = property on="Devices" class="MCListbox (strict)"("ItemNames"=w650) -> ()  [unwired: 2 in, 2 out]
        n185 = for {
          tunnel: w646 -> [w667]
          tunnel: Channel_States."Set Handle" ("State") -> [w666]
          tunnel: w656 -> [w665] mode=indexing
          tunnel: w657 -> [w662]
          tunnel: Channel_States."Measure" ("State") -> [w661]
          tunnel: w653 -> [w660]
          n186 = call-by-ref "?"(reference=w665, "OphirLMMeasurementLib.ICoLMMeasurement"=w662, "Handle in"=w667, "State"=w666) -> (reference out=w664:refnum<vi>, error out=w663:errorcluster)  [unwired: 8 in, 1 out]
          n187 = call-by-ref "?"(reference=w664, error in=w663, "Set Meas"=w660, "OphirLMMeasurementLib.ICoLMMeasurement"=w662, "State"=w661) -> ()  [unwired: 7 in, 3 out]
        }
      }
      event "Dev Control.UpdateInfo": Value Change {
        w669 = " - " ("string")
        n188 = event-data() -> ()  [unwired: 6 out]
        n189 = Unbundle By Name(w677) -> ("Devices"=w675:i32)
        n190 = Index Array(array=w676, index=w675) -> (element=w674:i32)
        n191 = invoke class="ICoLMMeasurement" method="GetDeviceInfo"(reference=w678, "hDevice"=w674) -> (error out=w673:errorcluster, "deviceName"=w672:string, "romVersion"=w671:string, "serialNumber"=w670:string)  [unwired: 5 in, 3 out]
        n192 = Concatenate Strings(w672, w669, w671, w669, w670) -> (→"Device Name":string)
      }
      event "Dev Control.ResetDev": Value Change {
        n193 = event-data() -> ()  [unwired: 2 out]
        n194 = Unbundle By Name(w687) -> ("Devices"=w679:i32)
        n195 = Index Array(array=w680, index=w679) -> (element=w683:i32)
        n196 = for {
          shift-right: [w693] -> w691
          shift-left: w692 -> [w693]
          tunnel: FALSE -> [w696]
          tunnel: Channel_States."Measure" ("State") -> [w695]
          tunnel: w688 -> [w694] mode=indexing
          # "Turn off\nMeasure-\nments"
          # "For each channel"
          n197 = call-by-ref "?"(reference=w694, "Set Meas"=w696, "OphirLMMeasurementLib.ICoLMMeasurement"=w693, "State"=w695) -> ()  [unwired: 8 in, 3 out]
        }
        n198 = invoke class="ICoLMMeasurement" method="ResetDevice"(reference=w691, "hDevice"=w683) -> (reference out=w686:refnum<k7>, error out=w685:errorcluster)  [unwired: 2 in, 2 out]
        n199 = Replace Array Subset(array=w680, new element=0 ("new element/subarray"), index=w679) -> (w681:i32[])
        n200 = local write "All Handles"(w681) -> ()
        n201 = invoke class="ICoLMMeasurement" method="Close"(reference=w686, error in=w685, "hDevice"=w683) -> (error out=w684:errorcluster)  [unwired: 1 in, 3 out]
      }
      event "Dev Control.ConfigCh", "Dev Control.Stream Modes:", "Dev Control.Value", "Dev Control.ExtTrig Window": Value Change {
        # "Don't do anything- Event loops need to handle changes of items changed\neven if they don't need to do anything with that change or the change won't\nbe used on the next iteration of the loop"
        n202 = event-data() -> ()  [unwired: 2 out]
      }
      event "Dev Control.SetConfig": Value Change {
        # "Sets the Channel, Stream Mode and Stream Mode Value for the current device"
        n203 = event-data() -> ()  [unwired: 2 out]
        n204 = Unbundle By Name(w702) -> ("Devices"=w706:i32)
        n205 = Index Array(array=w703, index=w706) -> (element=w707:i32)
        n206 = Unbundle By Name(w701) -> ("ConfigCh"=w700:i32, "Stream Modes:"=w699:i32, "Value"=w698:i32)
        n207 = invoke class="ICoLMMeasurement" method="ConfigureStreamMode"(reference=w705, "hDevice"=w707, "channel"=w700, "mode"=w699, "nValue"=w698) -> (error out=w704:errorcluster)  [unwired: 2 in, 6 out]
      }
      event "Dev Control.StartStream": Value Change {
        # "Start stream for all channels"
        n208 = event-data() -> ()  [unwired: 2 out]
        n209 = Unbundle By Name(w718) -> ("Devices"=w712:i32)
        n210 = Index Array(array=w717, index=w712) -> (element=w716:i32)
        n211 = for {
          tunnel: w719 -> [w727]
          tunnel: w716 -> [w723]
          tunnel: w715 -> [w722] mode=indexing
          tunnel: Channel_States."Measure" ("State") -> [w730]
          shift-right: [w728] -> w709
          shift-left: errorcluster {"status"=FALSE, "code"=0, "source"=""} ("error out") -> [w724]
          i -> [w721]
          n212 = invoke class="ICoLMMeasurement" method="IsSensorExists"(reference=w727, error in=w724, "hDevice"=w723, "channel"=w721) -> (reference out=w726:refnum<k7>, error out=w725:errorcluster, "exists"=w720:bool)  [unwired: 2 in, 3 out]
          n213 = case shown="True" w720 {
            tunnel: w721 -> [_ w738]
            tunnel: [w732 w737] -> w729
            tunnel: [w731 w736] -> w728
            tunnel: w726 -> [w732 w735]
            tunnel: w725 -> [w731 w734]
            tunnel: w723 -> [_ w733]
            frame False {
              # "Sensor doesn't exist, so skip"
            }
            frame True {
              n214 = invoke class="ICoLMMeasurement" method="StartStream"(reference=w735, error in=w734, "hDevice"=w733, "channel"=w738) -> (reference out=w737:refnum<k7>, error out=w736:errorcluster)  [unwired: 1 in, 3 out]
            }
          }
          n215 = call-by-ref "?"(reference=w722, "Set Meas"=w720, "OphirLMMeasurementLib.ICoLMMeasurement"=w729, "State"=w730) -> ()  [unwired: 8 in, 3 out]
        }
        n216 = Replace Array Subset(array=w713, new element=TRUE ("new element/subarray"), index=w712) -> (w710:bool[])
        n217 = local write "Meas On"(w710) -> ()
      }
      event "Dev Control.StopStream": Value Change {
        # "Stop stream for current channels"
        n218 = event-data() -> ()  [unwired: 2 out]
        n219 = Unbundle By Name(w746) -> ("Devices"=w748:i32)
        n220 = Index Array(array=w747, index=w748) -> (element=w739:i32)
        n221 = call "Stop All Channels streaming.vi"("Template Refs"=w743, "Handle"=w739, "LMMeasurementLib.ICoLMMeasurement"=w745) -> ("error out"=w744:errorcluster)
        n222 = Replace Array Subset(array=w740, new element=FALSE ("new element/subarray"), index=w739) -> (w741:bool[])
        n223 = local write "Meas On"(w741) -> ()
      }
      event "Dev Control.StopAll": Value Change {
        n224 = event-data() -> ()  [unwired: 2 out]
        n225 = Array Size(array=w753) -> (size(s)=w752:i32)
        n226 = Initialize Array(FALSE, w752) -> (w751:bool[])
        n227 = local write "Meas On"(w751) -> ()
        n228 = invoke class="ICoLMMeasurement" method="StopAllStreams"(reference=w758) -> (reference out=w755:refnum<k7>, error out=w749:errorcluster)  [unwired: 2 in, 1 out]
        n229 = for {
          tunnel: Channel_States."Measure" ("State") -> [w762]
          tunnel: w756 -> [w761] mode=indexing
          tunnel: w755 -> [w760]
          tunnel: FALSE -> [w759]
          # "Tells Channel Vis to stop measuring."
          n230 = call-by-ref "?"(reference=w761, "Set Meas"=w759, "OphirLMMeasurementLib.ICoLMMeasurement"=w760, "State"=w762) -> ()  [unwired: 8 in, 3 out]
        }
      }
      event "Dev Control.GetModes": Value Change {
        # "Gets External Trigger Modes from device and displays in externTrigModes"
        n231 = event-data() -> ()  [unwired: 2 out]
        n232 = Unbundle By Name(w771) -> ("Devices"=w769:i32)
        n233 = Index Array(array=w770, index=w769) -> (element=w768:i32)
        n234 = invoke class="ICoLMMeasurement" method="GetExtTrigModes"(reference=w772, "hDevice"=w768) -> (error out=w767:errorcluster, "index"=w764:i32, "options"=w765:variant)  [unwired: 4 in, 3 out]
        n235 = Variant To Data(type=string[] [], Variant=w765) -> (data=w763:string[])  [unwired: 1 in, 1 out]
        n236 = property on="externTrigModes" class="Ring (strict)"("Value"=w764, "Strings []"=w763) -> ()  [unwired: 2 in, 2 out]
      }
      event "Dev Control.externTrigModes": Value Change {
        # "Sets External Trigger Mode"
        n237 = event-data() -> ("NewVal"=w773:i32)  [unwired: 1 out]
        n238 = Unbundle By Name(w778) -> ("Devices"=w776:i32)
        n239 = Index Array(array=w777, index=w776) -> (element=w775:i32)
        n240 = invoke class="ICoLMMeasurement" method="SetExtTrigMode"(reference=w779, "hDevice"=w775, "index"=w773) -> (error out=w774:errorcluster)  [unwired: 2 in, 4 out]
      }
      event "Dev Control.GetWindow": Value Change {
        # "Gets External Trigger Window time from device and displays in extTrig Window"
        n241 = event-data() -> ()  [unwired: 2 out]
        n242 = Unbundle By Name(w785) -> ("Devices"=w783:i32)
        n243 = Index Array(array=w784, index=w783) -> (element=w782:i32)
        n244 = invoke class="ICoLMMeasurement" method="GetExtTrigWindowTime"(reference=w786, "hDevice"=w782) -> (error out=w781:errorcluster, "extTrigWindow"=w780:i32)  [unwired: 3 in, 3 out]
        n245 = property on="ExtTrig Window" class="DigNum (strict)"("Value"=w780) -> ()  [unwired: 2 in, 2 out]
      }
      event "Dev Control.Modify": Value Change {
        # "Set external trigger window time"
        n246 = event-data() -> ()  [unwired: 2 out]
        n247 = Unbundle By Name(w793) -> ("Devices"=w791:i32)
        n248 = Unbundle By Name(w788) -> ("ExtTrig Window"=w787:i32)
        n249 = Index Array(array=w792, index=w791) -> (element=w790:i32)
        n250 = invoke class="ICoLMMeasurement" method="SetExtTrigWindowTime"(reference=w794, "hDevice"=w790, "extTrigWindowTime"=w787) -> (error out=w789:errorcluster)  [unwired: 2 in, 4 out]
      }
      event "Read/Write.Write": Value Change {
        # "Writes the value in the Writestr control to the device.  If AutoRead = True, then it also reads from the device and displays the result in ReadStr"
        n251 = event-data() -> ()  [unwired: 2 out]
        n252 = Unbundle By Name(w804) -> ("Devices"=w802:i32)
        n253 = Unbundle By Name(w801) -> ("WriteStr"=w800:string, "AutoRead"=w799:bool)
        n254 = Index Array(array=w803, index=w802) -> (element=w795:i32)
        n255 = invoke class="ICoLMMeasurement" method="Write"(reference=w805, "hDevice"=w795, "command"=w800) -> (reference out=w798:refnum<k7>, error out=w797:errorcluster)  [unwired: 2 in, 3 out]
        n256 = case shown="True" w799 {
          tunnel: w798 -> [_ w811]
          tunnel: w797 -> [w806 w810]
          tunnel: [w806 w808] -> w796
          tunnel: w795 -> [_ w809]
          frame False {
          }
          frame True {
            n257 = invoke class="ICoLMMeasurement" method="Read"(reference=w811, error in=w810, "hDevice"=w809) -> (error out=w808:errorcluster, "reply"=→"ReadStr":string)  [unwired: 2 in, 3 out]
          }
        }
      }
      event "Read/Write.Read": Value Change {
        # "Reads from the device and displays the result in ReadStr"
        n258 = event-data() -> ()  [unwired: 2 out]
        n259 = Unbundle By Name(w818) -> ("Devices"=w816:i32)
        n260 = Index Array(array=w817, index=w816) -> (element=w814:i32)
        n261 = invoke class="ICoLMMeasurement" method="Read"(reference=w813, "hDevice"=w814) -> (error out=w815:errorcluster, "reply"=w812:string)  [unwired: 3 in, 3 out]
        n262 = local write "ReadStr"(w812) -> ()
      }
      event "Read/Write.AutoRead": Value Change {
        # "Don't do anything- Event loops need to handle changes of items changed\neven if they don't need to do anything with that change or the change won't\nbe used on the next iteration of the loop"
        n263 = event-data() -> ()  [unwired: 6 out]
      }
    }
    n264 = Unbundle By Name(w527) -> ("code"=w525:i32)
    n265 = Not Equal?(x=w528, y=w527) -> (x != y?=w526:bool)
    n266 = case shown="False" w526 {
      tunnel: w525 -> [w548 _]
      tunnel: w524 -> [w547 _]
      frame False {
        n267 = invoke class="ICoLMMeasurement" method="GetErrorFromCode"(reference=w547, "errorCode"=w548) -> ("errorString"=w540:string)  [unwired: 3 in, 4 out]
        "Last Error Code:" <- w540
        n268 = Equal?(x="No Error", y=w540) -> (x = y?=w541:bool)
        n269 = Empty String/Path?(string/path=w540) -> (empty?=w542:bool)
        n270 = Or(x=w541, y=w542) -> (x .or. y?=w543:bool)
        n271 = Select(t=u32 0, s=w543, f=u32 15667968) -> (s? t:f=w539:u32)
        n272 = property on="Last Error Code:" class="Str"("Text.FontColor"=w539) -> ()  [unwired: 2 in, 2 out]
      }
      frame True {
      }
    }
  }
  n273 = Obtain Queue(name (unnamed)="PM1_Queue", element data type=w25) -> (queue out=w13:refnum<queue>, error out=w21:errorcluster)  [unwired: 3 in, 1 out]
  n274 = Index Array(array=w22, index=0) -> (element=w6:refnum<event-registration>)
  n275 = Obtain Queue(name (unnamed)="PM2_Queue", element data type=w25) -> (queue out=w12:refnum<queue>, error out=w20:errorcluster)  [unwired: 3 in, 1 out]
  n276 = Index Array(array=w22, index=1) -> (element=w5:refnum<event-registration>)
  n277 = while {
    shift-right: [w824] -> w15
    shift-left: w6 -> [w822]
    tunnel: [w821] -> w8
    tunnel: w13 -> [w823]
    tunnel: [w826] -> w19
    tunnel: w21 -> [w827]
    tunnel: [w825] -> w18
    stop <- w821 stop-if-true
    n278 = local read "Stop"() -> (w821:bool)
    n279 = event shown="[0] <#1>: Value Change" {
      selector: w822 -> [_ _ _]
      dyn-events: [_ _ _] -> w824
      timeout: 1000 -> [_ _ _]
      tunnel: w823 -> [w832 w836 w838]
      tunnel: w827 -> [w831 w835 w837]
      tunnel: [w830 w836 w838] -> w826
      tunnel: [w829 w835 w837] -> w825
      tunnel: w821 -> [_ _ _]
      event Value Change {
        n280 = event-data() -> ("NewVal"=w828:variant)  [unwired: 1 in, 5 out]
        n281 = Variant To Data(type=T5 {"Value:"=[], " Time:"=[], " Status:"=[]} ("Ch1 Time/Status"), Variant=w828) -> (data=w833:T5)  [unwired: 1 in, 1 out]
        n282 = Enqueue Element(queue=w832, element=w833, error in (no error)=w831) -> (queue out=w830:refnum<queue>, error out=w829:errorcluster)  [unwired: 1 in, 1 out]
      }
      event "Stop": Value Change; Panel Close {
        n283 = event-data() -> ()  [unwired: 1 in, 3 out]
      }
      event Timeout {
        n284 = event-data() -> ()  [unwired: 1 in, 3 out]
      }
    }
  }
  n285 = while {
    shift-right: [w843] -> w14
    shift-left: w5 -> [w841]
    tunnel: [w840] -> w9
    tunnel: w12 -> [w842]
    tunnel: [w845] -> w17
    tunnel: w20 -> [w846]
    tunnel: [w844] -> w16
    stop <- w840 stop-if-true
    n286 = local read "Stop"() -> (w840:bool)
    n287 = event shown="[0] <#1>: Value Change" {
      selector: w841 -> [_ _ _]
      dyn-events: [_ _ _] -> w843
      timeout: 1000 -> [_ _ _]
      tunnel: w846 -> [w852 _ _]
      tunnel: w842 -> [w850 _ _]
      tunnel: [w849 _ _] -> w845
      tunnel: [w848 _ _] -> w844
      tunnel: w840 -> [_ _ _]
      event Value Change {
        n288 = event-data() -> ("NewVal"=w847:variant)  [unwired: 1 in, 5 out]
        n289 = Variant To Data(type=T5 {"Value:"=[], " Time:"=[], " Status:"=[]} ("Ch1 Time/Status"), Variant=w847) -> (data=w851:T5)  [unwired: 1 in, 1 out]
        n290 = Enqueue Element(queue=w850, element=w851, error in (no error)=w852) -> (queue out=w849:refnum<queue>, error out=w848:errorcluster)  [unwired: 1 in, 1 out]
      }
      event Panel Close; "Stop": Value Change {
        n291 = event-data() -> ()  [unwired: 1 in, 3 out]
      }
      event Timeout {
        n292 = event-data() -> ()  [unwired: 1 in, 3 out]
      }
    }
  }
  n293 = Unregister For Events(event registration refnum=w15) -> ()  [unwired: 1 in, 1 out]
  n294 = Release Queue(queue=w19, error in (no error)=w18) -> ()  [unwired: 1 in, 3 out]
  n295 = Release Queue(queue=w17, error in (no error)=w16) -> ()  [unwired: 1 in, 3 out]
  n296 = property class="App"() -> ("App.Kind"=w45:T6)  [unwired: 2 in, 2 out]
  n297 = Unregister For Events(event registration refnum=w14) -> ()  [unwired: 1 in, 1 out]
  n298 = Equal?(x=w45, y=w43) -> (x = y?=w40:bool)
  n299 = call "GenerateFilepathLA.vi"("Auto Date folder"=TRUE, "Filename"="Filename", "base path"="base path") -> ("operation (0:open)"=w32:T9, "file path"=w7:path)  [unwired: 1 in, 1 out]
  "file path" <- w7
  n300 = while {
    tunnel: [w857] -> w34
    tunnel: w7 -> [w854]
    stop <- w857 stop-if-true
    # "Check for filename changes and update file size"
    n301 = event shown="[1] \"Filename\", \"base path\": Value Change" {
      selector: _ -> [_ _]
      dyn-events: _ -> [_ _]
      timeout: 500 -> [_ _]
      event Timeout {
        n302 = event-data() -> ()  [unwired: 1 in, 3 out]
      }
      event "Filename", "base path": Value Change {
        n303 = event-data() -> ()  [unwired: 1 in, 6 out]
        n304 = flat-sequence {
          frame #0 {
            n305 = local read "TDMS error"() -> (w859:errorcluster)
            n306 = local read "TDMS file"() -> (w858:refnum<k34>)
            n307 = TDMS Close(8:w859, 11:w858) -> ()  [unwired: 2 out]
          }
          frame #1 {
            n308 = local read "Filename"() -> (w860:string)
            n309 = local read "base path"() -> (w866:path)
            n310 = call "GenerateFilepathLA.vi"("Auto Date folder"=TRUE, "Filename"=w860, "base path"=w866) -> ("operation (0:open)"=w863:T9, "file path"=w865:path)  [unwired: 1 in, 1 out]
            n311 = local write "file path"(w865) -> ()
            n312 = TDMS Open(10:w863, 11:w865) -> (0:w861:errorcluster, 3:w862:refnum<k34>)  [unwired: 5 in]
            n313 = local write "TDMS error"(w861) -> ()
            n314 = local write "TDMS file"(w862) -> ()
          }
        }
      }
    }
    n315 = File/Directory Info(path=w854) -> (size=→"File Size":i64)  [unwired: 1 in, 6 out]
    n316 = local read "Stop"() -> (w857:bool)
  }
  n317 = while {
    tunnel: w40 -> [w872]
    tunnel: w39 -> [_]
    tunnel: w34 -> [_]
    tunnel: w9 -> [_]
    tunnel: w8 -> [_]
    stop <- TRUE stop-if-true
    # "End program and reset stop button All wires make sure all the while loops have ended before running this loop"
    n318 = local read "TDMS error"() -> (w868:errorcluster)
    n319 = Quit LabVIEW(quit? (T)=w872) -> ()
    n320 = local read "TDMS file"() -> (w869:refnum<k34>)
    n321 = local write "Stop"(FALSE ("stop")) -> ()
    n322 = TDMS Close(8:w868, 11:w869) -> (0:w870:errorcluster)  [unwired: 1 out]
    n323 = call <vilib>:"Simple Error Handler.vi"("error in (no error)"=w870) -> ()  [unwired: 4 in, 5 out]
    "First Data point" <- TRUE
  }
  n324 = TDMS Open(10:w32, 11:w7) -> (0:→"TDMS error":errorcluster, 3:→"TDMS file":refnum<k34>)  [unwired: 5 in]
